vi "Label Targets3.vi"(7 "Annotate":bool=TRUE, 8 "Score Threshold":dbl, 9 "results":T1, 11 "Image in":T2) -> (3 "Image out":T2)   [LabVIEW 2023]
doc: "Draw scores near or on the particle and an ellipse around the target. Scores that are below the score threshold are drawn in red, above in green."
uses:
  <vilib>/vision/Image Controls.llb/IMAQ Image.ctl
  Target Fields.ctl
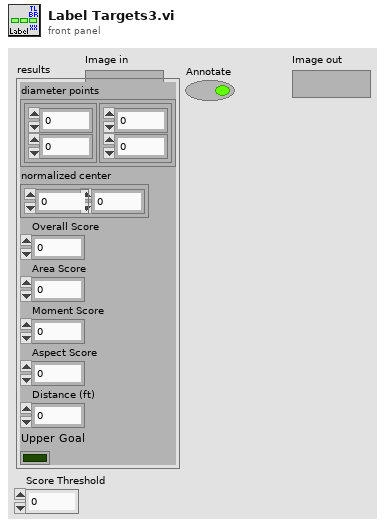
[diagram p1: front panel]
types:
  T1 = typedef "Target Fields.ctl" = cluster{"diameter points":cluster{"first point":cluster{"x":dbl, "y":dbl}, "projected point":cluster{"x":dbl, "y":dbl}}, "normalized center":cluster{"x":dbl, "y":dbl}, "Overall Score":dbl, "Area Score":dbl, "Moment Score":dbl, "Aspect Score":dbl, "Distance (ft)":dbl, "Upper Goal":bool}
  T2 = typedef "IMAQ Image.ctl" = refnum<image>
  T3 = cluster{"Desired Font (Application)":enum16{"User-specified Font", "Application Font", "System Font", "Dialog Font"}, "[User-specified Font]":cluster{"Font Name":string, "Size":i16, "Strikeout?":bool, "Italic?":bool, "Underline?":bool, "Outline?":bool, "Shadow?":bool, "Bold?":bool, "Rotation Angle":dbl}, "Horizontal Alignment":i16, "Vertical Alignment":i16}
  T4 = cluster{"first point":cluster{"x":dbl, "y":dbl}, "projected point":cluster{"x":dbl, "y":dbl}}
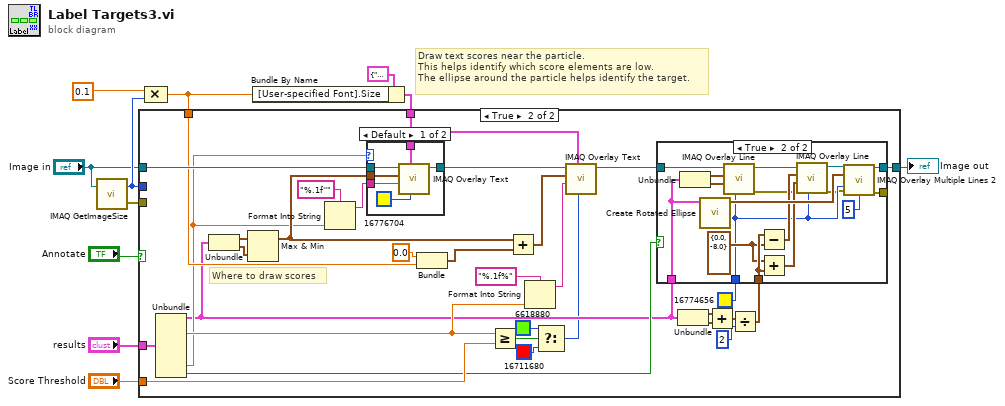
[diagram p0: block diagram]
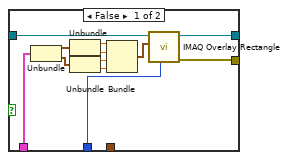
[diagram p3: hidden frame]
diagram:
  # "Draw text scores near the particle.\nThis helps identify which score elements are low.\nThe ellipse around the particle helps identify the target."
  n1 = call "IMAQ GetImageSize"("Image"="Image in") -> ("Y Resolution"=w8:i32, "error out"=w1:errorcluster)  [unwired: 3 in, 1 out]
  n2 = Compound Arithmetic op=MULTIPLY(0.1, w8) -> (w5:dbl)
  n3 = Bundle By Name(cluster=T3 {"Desired Font (Application)"=enum."User-specified Font", "[User-specified Font]"={"Font Name"="Ariel", "Size"=12, "Strikeout?"=FALSE, "Italic?"=FALSE, "Underline?"=FALSE, "Outline?"=FALSE, "Shadow?"=FALSE, "Bold?"=FALSE, "Rotation Angle"=0.0}, "Horizontal Alignment"=0, "Vertical Alignment"=0} ("Font, Size & Style"), "[User-specified Font].Size"=w5) -> (w6:T3)
  n4 = case shown="True" "Annotate" {
    tunnel: [w12 w38] -> w11
    tunnel: "Image in" -> [w12 w44]
    tunnel: w6 -> [_ w28]
    tunnel: w8 -> [_ _]
    tunnel: w5 -> [_ w40]
    tunnel: "results" -> [_ w39]
    tunnel: "Score Threshold" -> [_ w30]
    tunnel: w1 -> [_ _]
    frame False {
    }
    frame True {
      # "Where to draw scores"
      n5 = Unbundle(w39) -> ("diameter points"=w25:T4, "Overall Score"=w37:dbl, "Distance (ft)"=w29:dbl, "Upper Goal"=w27:bool)  [unwired: 4 out]
      n6 = Unbundle(w25) -> ("first point"=w32:cluster{"x":dbl, "y":dbl}, "projected point"=w33:cluster{"x":dbl, "y":dbl})
      n7 = Max & Min(x=w32, y=w33) -> (max(x,y)=w31:cluster{"x":dbl, "y":dbl})  [unwired: 1 out]
      n8 = Format Into String(format string="%.1f''", w29) -> (resulting string=w43:string)  [unwired: 2 in, 1 out]
      n9 = case shown="Default" w29 {
        tunnel: w44 -> [w79 w80]
        tunnel: w43 -> [w78 _]
        tunnel: w28 -> [w77 _]
        tunnel: [w76 w80] -> w36
        tunnel: w31 -> [w75 _]
        frame Default {
          n10 = call "IMAQ Overlay Text"("Text Color (black)"=u32 16776704 ("Color"), "Font, Size & Style"=w77, "String"=w78, "Origin"=w75, "Image"=w79) -> ("Image Out"=w76:T2)  [unwired: 5 in, 1 out]
        }
        frame 0 {
        }
      }
      n11 = Bundle(0.0, w40) -> (w34:cluster{dbl, dbl})  [unwired: 1 in]
      n12 = Greater Or Equal?(x=w37, y=w30) -> (x >= y?=w13:bool)
      n13 = Add(x=w31, y=w34) -> (x+y=w17:cluster{dbl, dbl})
      n14 = Format Into String(format string="%.1f%", w37) -> (resulting string=w18:string)  [unwired: 2 in, 1 out]
      n15 = Select(t=u32 6618880 ("Color"), s=w13, f=u32 16711680 ("Color")) -> (s? t:f=w14:u32)
      n16 = call "IMAQ Overlay Text"("Text Color (black)"=w14, "Font, Size & Style"=w28, "String"=w18, "Origin"=w17, "Image"=w36) -> ("Image Out"=w35:T2)  [unwired: 5 in, 1 out]
      n17 = Unbundle(w25) -> ("first point"=w24:cluster{"x":dbl, "y":dbl}, "projected point"=w23:cluster{"x":dbl, "y":dbl})
      n18 = Add(x=w24, y=w23) -> (x+y=w22:cluster{"x":dbl, "y":dbl})
      n19 = Divide(x=w22, y=u32 2 ("Width")) -> (x/y=w20:cluster{"x":dbl, "y":dbl})
      n20 = case shown="True" w27 {
        tunnel: [w55 w71] -> w38
        tunnel: w25 -> [w53 w68]
        tunnel: w35 -> [w56 w67]
        tunnel: u32 16774656 ("Color") -> [w54 w60]
        tunnel: w20 -> [_ w64]
        tunnel: [w45 w57] -> _
        frame False {
          n21 = Unbundle(w53) -> ("first point"=w52:cluster{"x":dbl, "y":dbl}, "projected point"=w51:cluster{"x":dbl, "y":dbl})
          n22 = Unbundle(w52) -> ("x"=w50:dbl, "y"=w49:dbl)
          n23 = Unbundle(w51) -> ("x"=w48:dbl, "y"=w47:dbl)
          n24 = Bundle("x"=w50, "y"=w49, "x"=w48, "y"=w47) -> (w46:cluster{"x":dbl, "y":dbl, "x":dbl, "y":dbl})  [unwired: 1 in]
          n25 = call "IMAQ Overlay Rectangle"("Color"=w54, "Rectangle"=w46, "Image"=w56) -> ("error out"=w45:errorcluster, "Image Out"=w55:T2)  [unwired: 7 in]
        }
        frame True {
          w61 = cluster{"x":dbl, "y":dbl} {"x"=0.0, "y"=-8.0} ("x/y")
          n26 = Unbundle(w68) -> ("first point"=w73:cluster{"x":dbl, "y":dbl}, "projected point"=w72:cluster{"x":dbl, "y":dbl})
          n27 = call "Create Rotated Ellipse.vi"("diameter points"=w68) -> ("XY Graph"=w70:cluster{"X":dbl, "Y":dbl}[])  [unwired: 10 in]
          n28 = call "IMAQ Overlay Line"("Color"=w60, "End Point"=w72, "Start Point"=w73, "Image"=w67) -> ("error out"=w59:errorcluster, "Image Out"=w66:T2)  [unwired: 6 in]
          n29 = Subtract(x=w64, y=w61) -> (x-y=w63:cluster{"x":dbl, "y":dbl})
          n30 = Add(x=w61, y=w64) -> (x+y=w62:cluster{"x":dbl, "y":dbl})
          n31 = call "IMAQ Overlay Line"("Color"=w60, "error in (no error)"=w59, "End Point"=w62, "Start Point"=w63, "Image"=w66) -> ("error out"=w58:errorcluster, "Image Out"=w65:T2)  [unwired: 5 in]
          n32 = call "IMAQ Overlay Multiple Lines 2"("Image"=w65, "Line End Points"=w70, "Color"=w60, "error in (no error)"=w58, "Width"=u32 5) -> ("Image Out"=w71:T2, "error out"=w57:errorcluster)  [unwired: 9 in]
        }
      }
    }
  }
  "Image out" <- w11
